vi "CRYChannel Table.vi"(1 "I_Device Info":T3(array[cluster]), 2 "I_Channel Info":T4[](array[typedef]) {"Coupling" items=["Default"=-1, "RSE"=10083, "NRSE"=10078, "Differential"=10106, "Pseudodifferential"=12529]; "term config" items=["Default"=-1, "RSE"=10083, "NRSE"=10078, "Differential"=10106, "Pseudodifferential"=12529]; "Anti-aliasing Factor (%fs)" format="%.2f"}, 7 "I_Name In":string[][](array[string]), 9 "O_Name In":string[][](array[string]), 12 "O_Device Info":T3(array[cluster]), 13 "O_Channel Info":T4[](array[typedef]) {"Coupling" items=["Default"=-1, "RSE"=10083, "NRSE"=10078, "Differential"=10106, "Pseudodifferential"=12529]; "term config" items=["Default"=-1, "RSE"=10083, "NRSE"=10078, "Differential"=10106, "Pseudodifferential"=12529]; "Anti-aliasing Factor (%fs)" format="%.2f"}) -> (4 "O_Channel Info Out":T4[](array[typedef]) {"Coupling" items=["Default"=-1, "RSE"=10083, "NRSE"=10078, "Differential"=10106, "Pseudodifferential"=12529]; "term config" items=["Default"=-1, "RSE"=10083, "NRSE"=10078, "Differential"=10106, "Pseudodifferential"=12529]; "Anti-aliasing Factor (%fs)" format="%.2f"}, 6 "I_Channel Info Out":T4[](array[typedef]) {"Coupling" items=["Default"=-1, "RSE"=10083, "NRSE"=10078, "Differential"=10106, "Pseudodifferential"=12529]; "term config" items=["Default"=-1, "RSE"=10083, "NRSE"=10078, "Differential"=10106, "Pseudodifferential"=12529]; "Anti-aliasing Factor (%fs)" format="%.2f"}, 8 "I_Name Out":string[][](array[string]), 10 "O_Name Out":string[][](array[string]), 15 "Return Flag":bool)   [LabVIEW 2013]
uses:
  Typedef Control/CRYHardware Channel Info.ctl
  <vilib>/Utility/miscctls.llb/LVBoundsTypeDef.ctl
  <vilib>/Utility/miscctls.llb/LVPositionTypeDef.ctl
  <vilib>/Utility/miscctls.llb/LVStringsAndValuesArrayTypeDef.ctl
panel:
  in  "Out_In Old":bool
  out "Row Old":i32
  out "Column Old":i32
  in  "Update":bool
  out "SelectValue":u32
  out "Device Name":string
  out "Cell Position":T1
  out "Cell Size":T2
  out "Column":i32
  out "Row":i32
  in  "Out_In":bool
  in  "SelectSate":bool
  in  "VmaxText":string
  in  "SelectRing":u32(ring) items=["8 bit"=8, "16 bit"=16, "24 bit"=24, "32 bit"=32]
  in  "I_MList":i32(listbox) caption="Input Channels"
  in  "I_Duplicate":bool
  in  "I_Delete":bool
  in  "I_Add":bool
  in  "O_Duplicate":bool
  in  "O_Delete":bool
  in  "O_Add":bool
  in  "Cancel":bool
  in  "OK":bool
  in  "O_MList":i32[](listbox) caption="Output Channels"
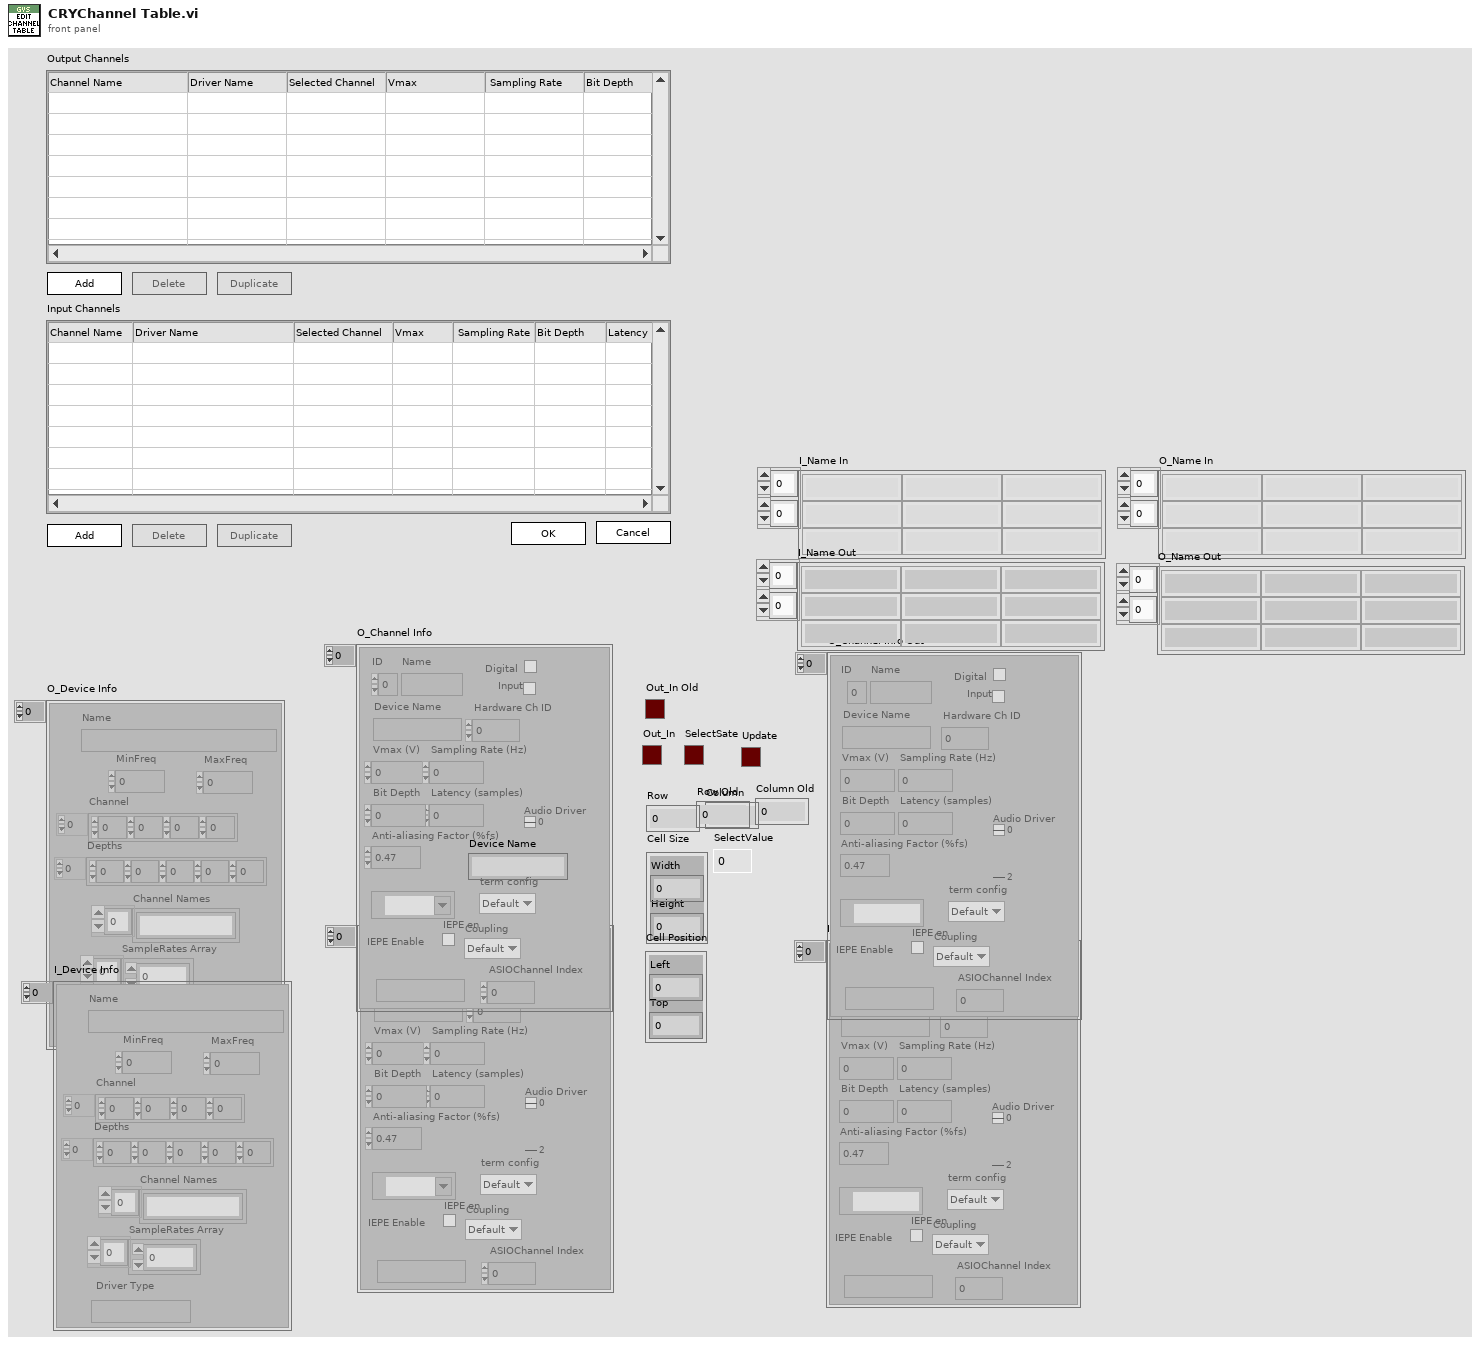
[diagram p1: front panel]
types:
  T1 = typedef "LVPositionTypeDef.ctl" = cluster{"Left":i32, "Top":i32}
  T2 = typedef "LVBoundsTypeDef.ctl" = cluster{"Width":u32, "Height":u32}
  T3 = cluster{"Name":string, "MinFreq":dbl, "MaxFreq":dbl, "Channel":i32[], "Depths":i32[], "Channel Names":string[], "SampleRates Array":dbl[], "Driver Type":string}[]
  T4 = typedef "CRYHardware Channel Info.ctl" = cluster{"ID":i32, "Name":string, "Digital":bool, "Input":bool, "Device Name":string, "Hardware Ch ID":u8, "Vmax (V)":dbl, "Latency (samples)":dbl, "Sampling Rate (Hz)":u32, "Bit Depth":u32, "Anti-aliasing Factor (%fs)":sgl, "DAQmx Channel":tag, "term config":i32, "Coupling":i32, "IEPE en":bool, "ASIOChannel Name":string, "Audio Driver":u16, "ASIOChannel Index":u8}
  T5 = typedef "LVStringsAndValuesArrayTypeDef.ctl" = cluster{"String":string, "Value":ext}[]
  T6 = typedef "LVPoint32TypeDef.ctl" = cluster{"Horizontal":i32, "Vertical":i32}
  T7 = typedef "LVRowAndColumnTypeDef.ctl" = cluster{"Row":i32, "Column":i32}
  T8 = cluster{"Name":string, "MinFreq":dbl, "MaxFreq":dbl, "Channel":i32[], "Depths":i32[], "Channel Names":string[], "SampleRates Array":dbl[], "Driver Type":string}
  T9 = cluster{"O_Add":bool, "O_Delete":bool, "O_Duplicate":bool, "I_Add":bool, "I_Delete":bool, "I_Duplicate":bool, "Update":bool}
  T10 = cluster{"Name":string, "Device Name":string, "Device Name":string, string, string, string}
  T11 = cluster{"Name":string, "Device Name":string, "Device Name":string, string, string, string, string}
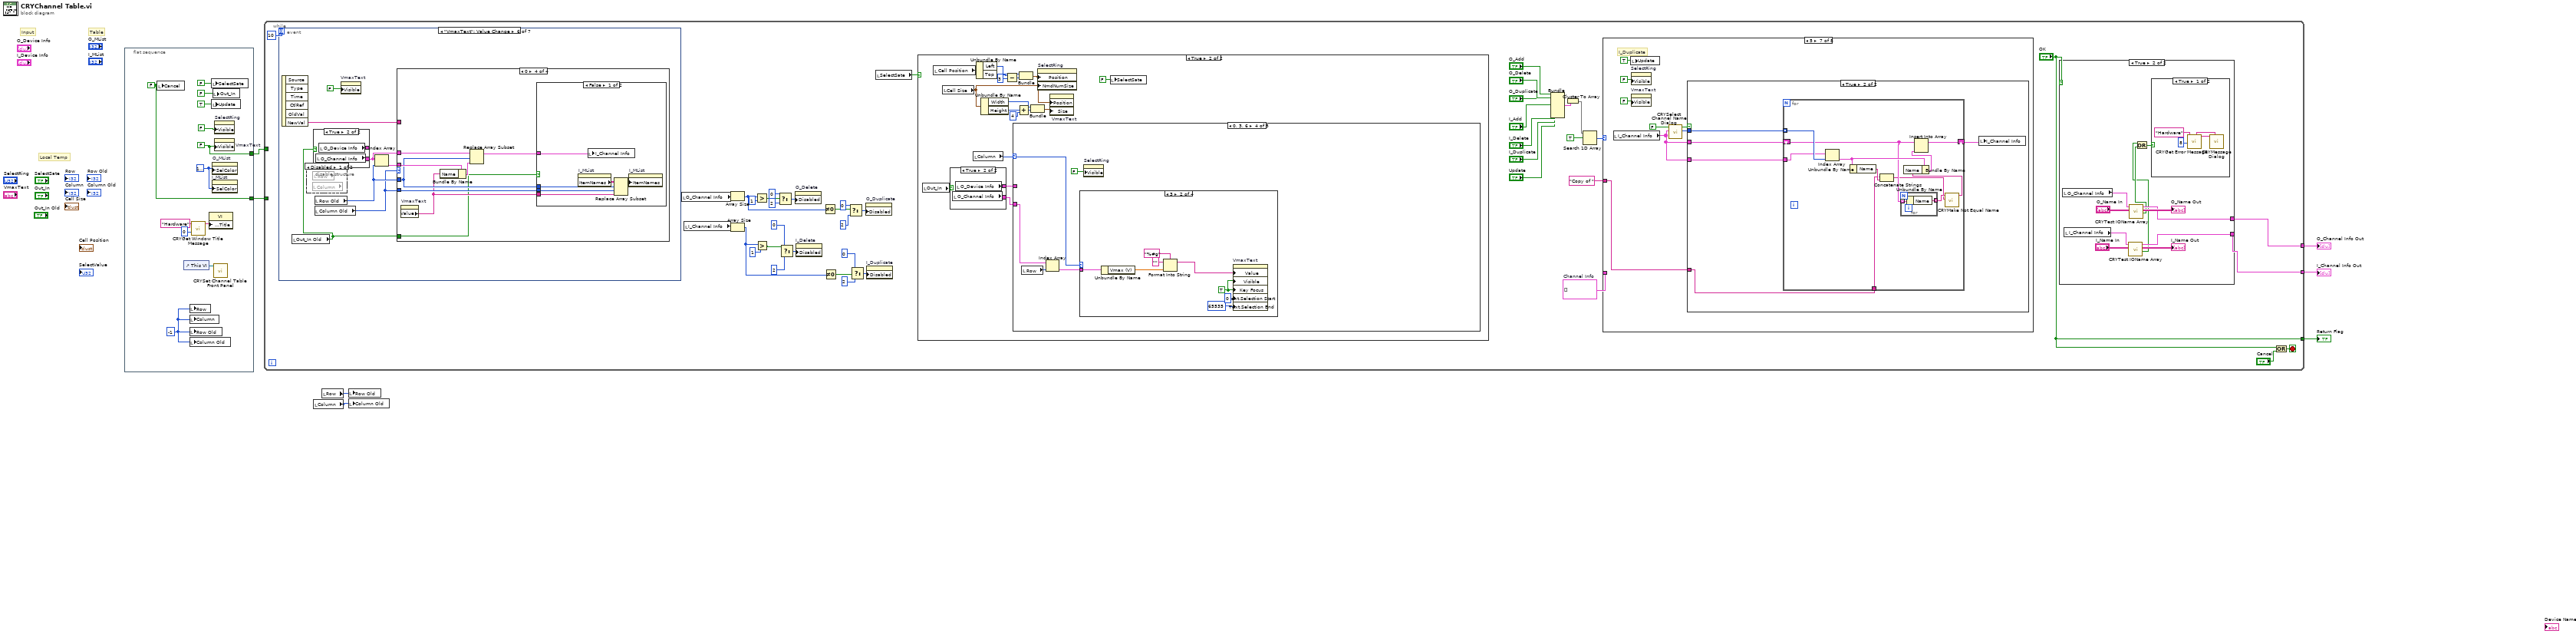
[diagram p0: block diagram]
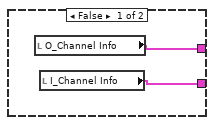
[diagram p2: hidden frame]
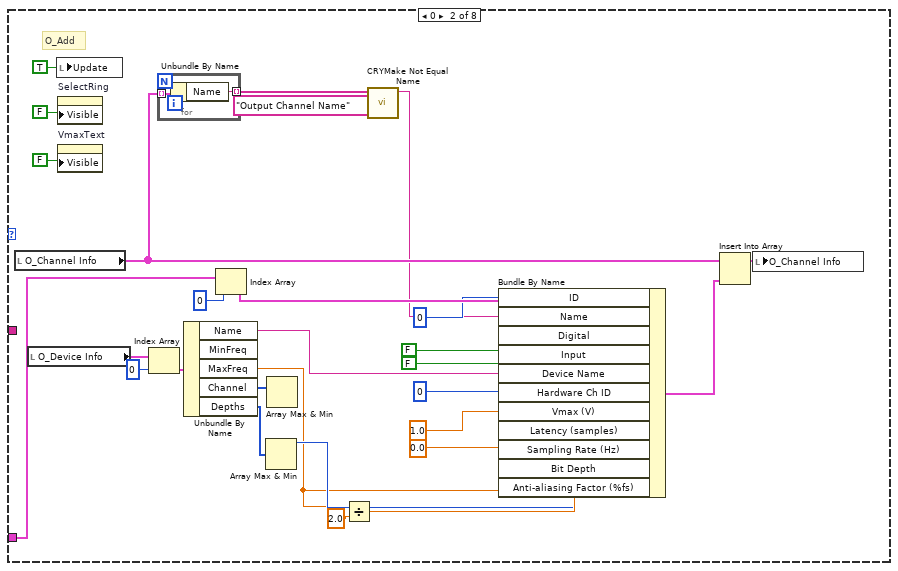
[diagram p5: hidden frame]
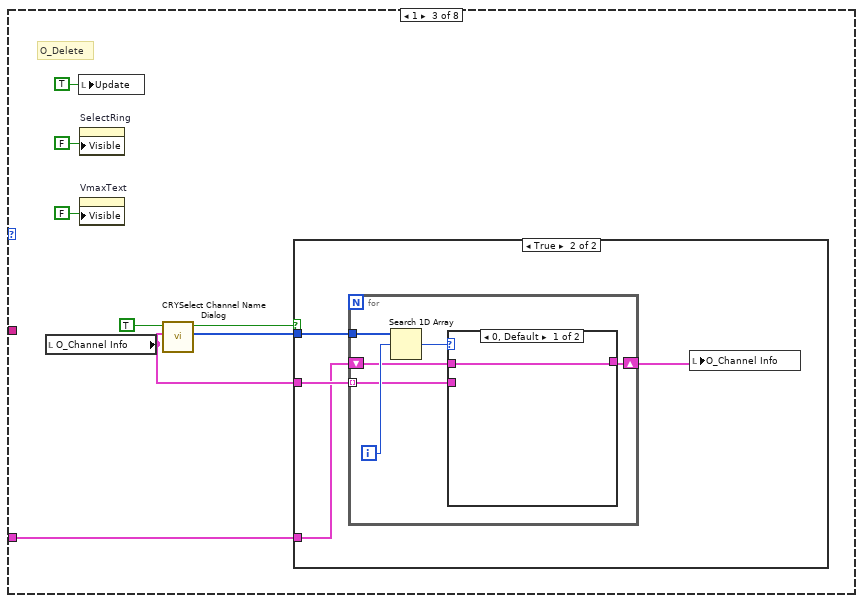
[diagram p6: hidden frame]
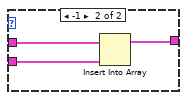
[diagram p8: hidden frame]
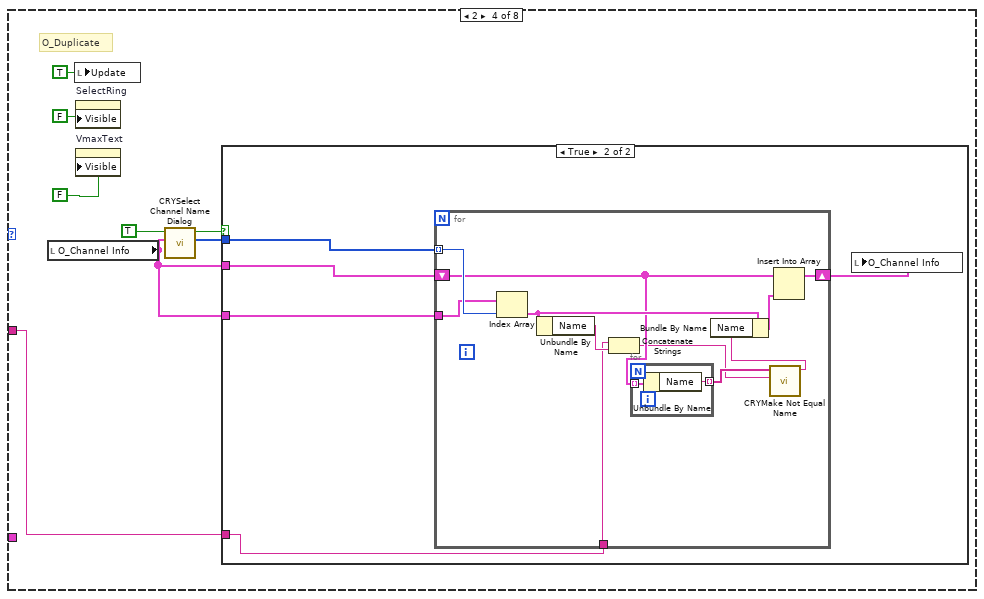
[diagram p9: hidden frame]
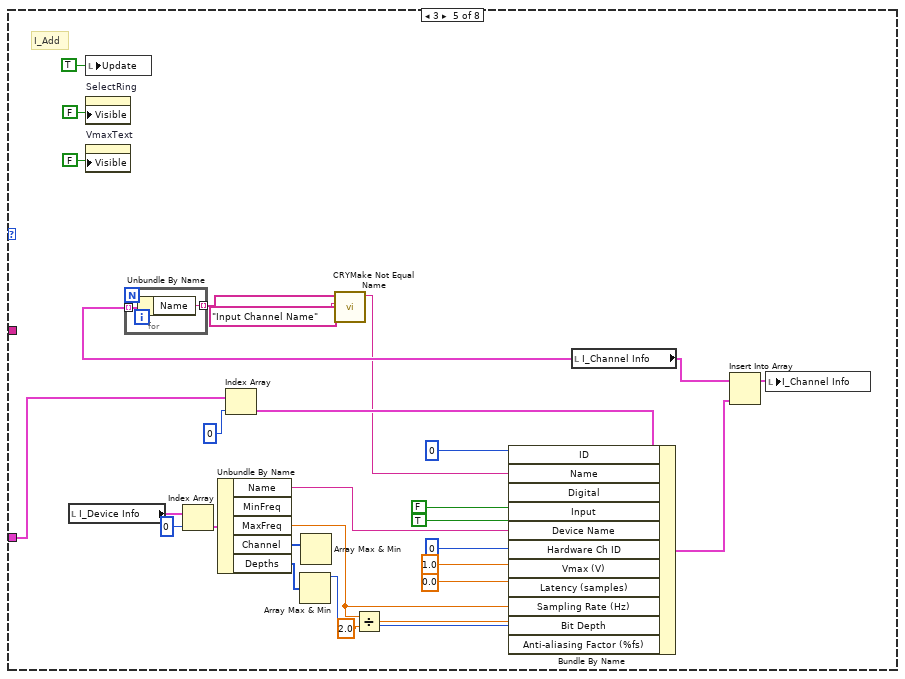
[diagram p11: hidden frame]
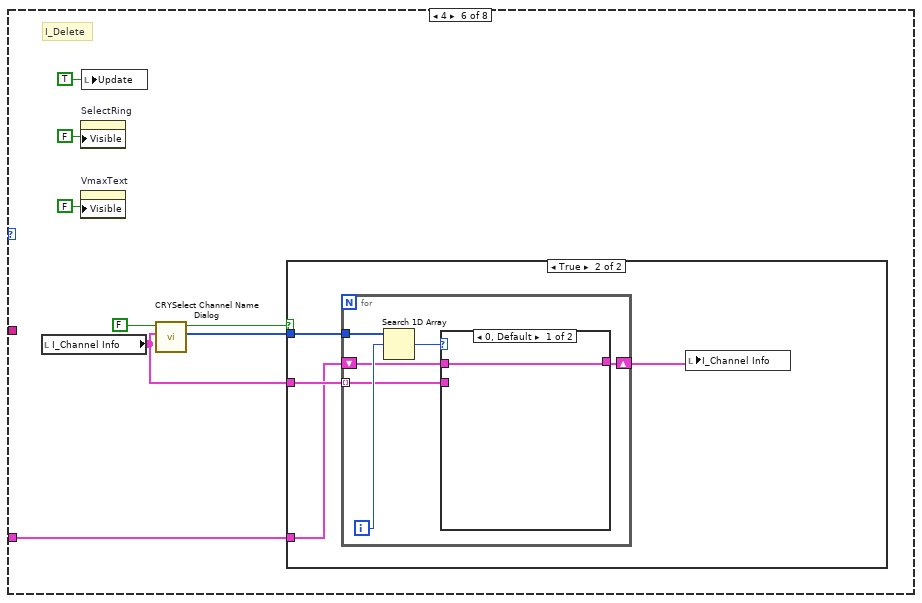
[diagram p12: hidden frame]
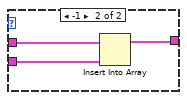
[diagram p14: hidden frame]
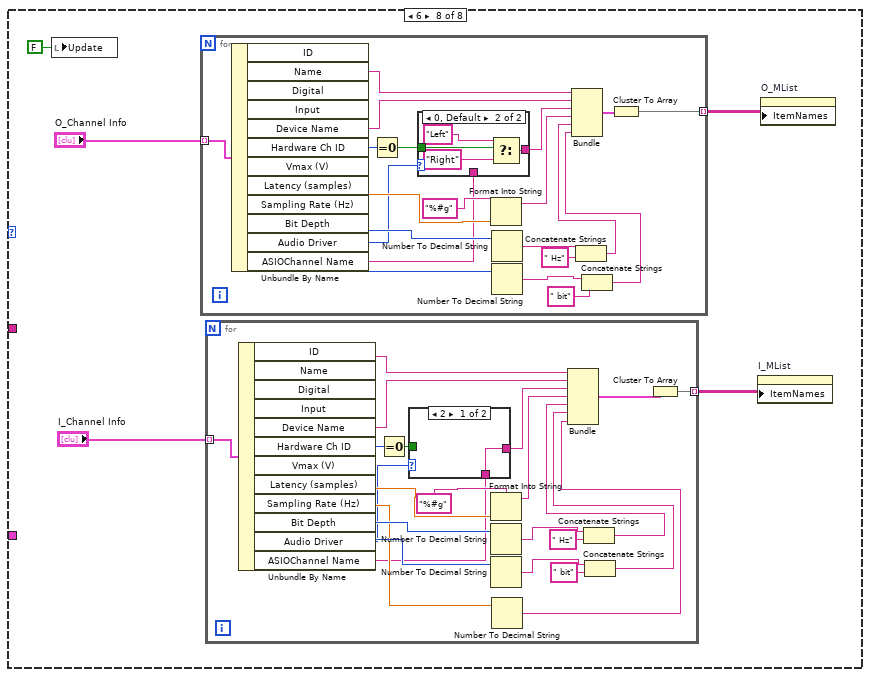
[diagram p16: hidden frame]
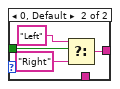
[diagram p17: hidden frame]
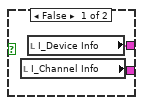
[diagram p20: hidden frame]
diagram:
  # "Table"
  # "Input"
  # "Local Temp"
  n1 = flat-sequence {
    tunnel: [w14] -> w4
    tunnel: [w9] -> w3
    frame #0 {
      w8 = -1 ("Row Old")
      w9 = FALSE ("Cancel")
      w15 = u32 16777226
      w14 = FALSE ("Visible")
      n2 = local write "Cancel"(w9) -> ()
      n3 = control-ref of="This VI"() -> (w10:refnum<vi>)
      n4 = local write "Row"(w8) -> ()
      n5 = local write "Column"(w8) -> ()
      n6 = local write "Row Old"(w8) -> ()
      n7 = local write "Column Old"(w8) -> ()
      n8 = call "CRYGet Window Title Message.vi"("No"=0 ("Error No"), "Kind"="Hardware") -> ("Multibyte String"=w13:string)  [unwired: 4 in, 5 out]
      n9 = property class="VI"("Front Panel.Title"=w13) -> ()  [unwired: 2 in, 2 out]
      n10 = local write "SelectSate"(FALSE ("SelectSate")) -> ()
      n11 = local write "Update"(TRUE ("Update")) -> ()
      n12 = property on="O_MList" class="MCListbox (strict)"("SelColor"=w15) -> ()  [unwired: 2 in, 2 out]
      n13 = property on="I_MList" class="MCListbox (strict)"("SelColor"=w15) -> ()  [unwired: 2 in, 2 out]
      n14 = local write "Out_In"(FALSE ("Out/In")) -> ()
      n15 = call "CRYSet Channel Table Front Panel.vi"("Vi Ref"=w10) -> ()  [unwired: 11 in]
      n16 = property on="SelectRing" class="Ring (strict)"("Visible"=FALSE) -> ()  [unwired: 2 in, 2 out]
      n17 = property on="VmaxText" class="Str"("Visible"=w14) -> ()  [unwired: 2 in, 2 out]
    }
  }
  n18 = while {
    tunnel: ["OK"] -> w7
    tunnel: [w21] -> w6
    tunnel: [w20] -> w5
    tunnel: w4 -> [_]
    tunnel: w3 -> [_]
    stop <- w61 stop-if-true
    w47 = T4[] []  # Channel Info
    n19 = event shown="[5] \"VmaxText\": Value Change" {
      selector: _ -> [_ _ _ _ _ _ _]
      dyn-events: _ -> [_ _ _ _ _ _ _]
      timeout: 10 -> [_ _ _ _ _ _ _]
      event Timeout {
        n20 = event-data() -> ()  [unwired: 3 out]
      }
      event "O_MList": Mouse Down {
        n21 = event-data() -> ("Coords"=w484:T6)  [unwired: 8 out]
        n22 = flat-sequence {
          tunnel: w477 -> [w497]
          tunnel: [w497] -> w476
          frame #0 {
            n23 = local read "Column"() -> (w499:i32)
            n24 = local read "Row"() -> (w498:i32)
            n25 = local write "Row Old"(w498) -> ()
            n26 = local write "Column Old"(w499) -> ()
          }
        }
        n27 = invoke on="O_MList" class="MCListbox (strict)" method="Point To Row Column"("Point"=w484) -> ("CellPosition"=w477:T7)  [unwired: 6 in, 6 out]
        n28 = local read "Row"() -> (w475:i32)
        n29 = case shown="0, Default" w475 {
          frame 0, Default {
            n30 = flat-sequence {
              frame #0 {
                n31 = local read "Out_In"() -> (w494:bool)
                n32 = local write "Out_In Old"(w494) -> ()
              }
              frame #1 {
                n33 = local write "Out_In"(TRUE ("Out/In")) -> ()
              }
            }
          }
          frame -1 {
            w496 = TRUE ("Out/In")
            n34 = local write "Out_In"(w496) -> ()
            n35 = local write "Out_In Old"(w496) -> ()
          }
        }
        n36 = property on="O_MList" class="MCListbox (strict)"("ActiveCell"=w476) -> ("CellSize"=w481:T2, "ActiveCellPos"=w482:T1)  [unwired: 2 in, 2 out]
        n37 = Unbundle By Name(w476) -> ("Row"=w479:i32, "Column"=w480:i32)
        n38 = local read "O_Channel Info"() -> (w493:T4[])
        n39 = local write "Cell Size"(w481) -> ()
        n40 = local write "Cell Position"(w482) -> ()
        n41 = Equal To 0?(x=w479) -> (x = 0?=w486:bool)
        n42 = Equal To 0?(x=w480) -> (x = 0?=w485:bool)
        n43 = local write "Row"(w479) -> ()
        n44 = local write "Column"(w480) -> ()
        n45 = Compound Arithmetic op=AND(w486, w485) -> (w478:bool)
        n46 = Array Size(array=w493) -> (size(s)=w492:i32)
        n47 = case shown="True" w478 {
          tunnel: w482 -> [_ w514]
          tunnel: w484 -> [_ w515]
          tunnel: w481 -> [_ w513]
          tunnel: [TRUE w501] -> w483
          frame False {
          }
          frame True {
            n48 = Unbundle By Name(w515) -> ("Horizontal"=w506:i32, "Vertical"=w510:i32)
            n49 = Unbundle By Name(w513) -> ("Width"=w512:u32, "Height"=w511:u32)
            n50 = Unbundle By Name(w514) -> ("Left"=w504:i32, "Top"=w502:i32)
            n51 = Add(x=w504, y=w512) -> (x+y=w505:u32)
            n52 = Add(x=w502, y=w511) -> (x+y=w503:u32)
            n53 = In Range and Coerce(upper limit=w505, x=w506, lower limit=w504) -> (In Range?=w509:bool)  [unwired: 1 out]
            n54 = In Range and Coerce(upper limit=w503, x=w510, lower limit=w502) -> (In Range?=w508:bool)  [unwired: 1 out]
            n55 = Compound Arithmetic op=AND(w509, w508) -> (w507:bool)
            n56 = case shown="True" w507 {
              tunnel: [FALSE TRUE] -> w501
              frame False {
              }
              frame True {
              }
            }
          }
        }
        n57 = Less?(x=w479, y=w492) -> (x < y?=w491:bool)
        n58 = Greater Or Equal?(x=w479, y=0) -> (x >= y?=w490:bool)
        n59 = Build Array(w491, w490, w483) -> (w489:bool[])
        n60 = And Array Elements(Boolean array=w489) -> (logical AND=w488:bool)
        n61 = local write "SelectSate"(w488) -> ()
        n62 = case shown="False" w488 {
          frame False {
            n63 = property on="VmaxText" class="Str"("Visible"=FALSE) -> ()  [unwired: 2 in, 2 out]
            n64 = property on="SelectRing" class="Ring (strict)"("Visible"=FALSE) -> ()  [unwired: 2 in, 2 out]
          }
          frame True {
          }
        }
      }
      event "O_MList", "I_MList": Mouse Move {
        n65 = event-data() -> ("Coords"=w528:T6)  [unwired: 5 out]
        n66 = invoke on="O_MList" class="MCListbox (strict)" method="Point To Row Column"("Point"=w528) -> ("CellPosition"=w527:T7)  [unwired: 6 in, 6 out]
        n67 = Unbundle By Name(w527) -> ("Row"=w524:i32, "Column"=w526:i32)
        n68 = local read "Column"() -> (w525:i32)
        n69 = local read "Row"() -> (w523:i32)
        n70 = Not Equal?(x=w526, y=w525) -> (x != y?=w521:bool)
        n71 = Not Equal?(x=w524, y=w523) -> (x != y?=w522:bool)
        n72 = Or(x=w522, y=w521) -> (x .or. y?=w520:bool)
        n73 = case shown="True" w520 {
          frame True {
            n74 = property on="SelectRing" class="Ring (strict)"("Visible"=FALSE) -> ()  [unwired: 2 in, 2 out]
          }
          frame False {
          }
        }
      }
      event "I_MList": Mouse Down {
        n75 = event-data() -> ("Coords"=w533:T6)  [unwired: 8 out]
        n76 = flat-sequence {
          tunnel: w532 -> [w553]
          tunnel: [w553] -> w531
          frame #0 {
            n77 = local read "Column"() -> (w555:i32)
            n78 = local read "Row"() -> (w554:i32)
            n79 = local write "Row Old"(w554) -> ()
            n80 = local write "Column Old"(w555) -> ()
          }
        }
        n81 = invoke on="I_MList" class="MCListbox (strict)" method="Point To Row Column"("Point"=w533) -> ("CellPosition"=w532:T7)  [unwired: 6 in, 6 out]
        n82 = local read "Row"() -> (w530:i32)
        n83 = local read "I_Channel Info"() -> (w549:T4[])
        n84 = property on="I_MList" class="MCListbox (strict)"("ActiveCell"=w531) -> ("CellSize"=w538:T2, "ActiveCellPos"=w539:T1)  [unwired: 2 in, 2 out]
        n85 = Unbundle By Name(w531) -> ("Row"=w535:i32, "Column"=w536:i32)
        n86 = case shown="0, Default" w530 {
          frame 0, Default {
            n87 = flat-sequence {
              frame #0 {
                n88 = local read "Out_In"() -> (w550:bool)
                n89 = local write "Out_In Old"(w550) -> ()
              }
              frame #1 {
                n90 = local write "Out_In"(FALSE ("Out/In")) -> ()
              }
            }
          }
          frame -1 {
            w552 = FALSE ("Out/In")
            n91 = local write "Out_In"(w552) -> ()
            n92 = local write "Out_In Old"(w552) -> ()
          }
        }
        n93 = Equal To 0?(x=w535) -> (x = 0?=w541:bool)
        n94 = Equal To 0?(x=w536) -> (x = 0?=w540:bool)
        n95 = local write "Column"(w536) -> ()
        n96 = local write "Cell Position"(w539) -> ()
        n97 = local write "Row"(w535) -> ()
        n98 = local write "Cell Size"(w538) -> ()
        n99 = Compound Arithmetic op=AND(w541, w540) -> (w534:bool)
        n100 = Array Size(array=w549) -> (size(s)=w548:i32)
        n101 = Less?(x=w535, y=w548) -> (x < y?=w545:bool)
        n102 = Greater Or Equal?(x=w535, y=0) -> (x >= y?=w544:bool)
        n103 = Greater Or Equal?(x=w536, y=1) -> ()  [unwired: 1 out]
        n104 = case shown="True" w534 {
          tunnel: w539 -> [_ w570]
          tunnel: w533 -> [_ w571]
          tunnel: w538 -> [_ w569]
          tunnel: [TRUE w557] -> w537
          frame False {
          }
          frame True {
            n105 = Unbundle By Name(w571) -> ("Horizontal"=w562:i32, "Vertical"=w566:i32)
            n106 = Unbundle By Name(w569) -> ("Width"=w568:u32, "Height"=w567:u32)
            n107 = Unbundle By Name(w570) -> ("Left"=w560:i32, "Top"=w558:i32)
            n108 = Add(x=w560, y=w568) -> (x+y=w561:u32)
            n109 = Add(x=w558, y=w567) -> (x+y=w559:u32)
            n110 = In Range and Coerce(upper limit=w561, x=w562, lower limit=w560) -> (In Range?=w565:bool)  [unwired: 1 out]
            n111 = In Range and Coerce(upper limit=w559, x=w566, lower limit=w558) -> (In Range?=w564:bool)  [unwired: 1 out]
            n112 = Compound Arithmetic op=AND(w565, w564) -> (w563:bool)
            n113 = case shown="False" w563 {
              tunnel: [FALSE TRUE] -> w557
              frame False {
              }
              frame True {
              }
            }
          }
        }
        n114 = Build Array(w545, w544, w537) -> (w543:bool[])
        n115 = And Array Elements(Boolean array=w543) -> (logical AND=w542:bool)
        n116 = case shown="False" w542 {
          frame False {
            n117 = property on="VmaxText" class="Str"("Visible"=FALSE) -> ()  [unwired: 2 in, 2 out]
            n118 = property on="SelectRing" class="Ring (strict)"("Visible"=FALSE) -> ()  [unwired: 2 in, 2 out]
          }
          frame True {
          }
        }
        n119 = local write "SelectSate"(w542) -> ()
      }
      event "SelectRing": Value Change {
        n120 = event-data() -> ("NewVal"=w578:u32)  [unwired: 6 out]
        n121 = local read "Out_In"() -> (w583:bool)
        n122 = case shown="False" w583 {
          tunnel: [w699 w701] -> w579
          tunnel: [w698 w700] -> w580
          frame False {
            n123 = local read "I_Channel Info"() -> (w699:T4[])
            n124 = local read "I_Device Info"() -> (w698:T3)
          }
          frame True {
            n125 = local read "O_Channel Info"() -> (w701:T4[])
            n126 = local read "O_Device Info"() -> (w700:T3)
          }
        }
        n127 = local write "Update"(TRUE ("Update")) -> ()
        n128 = local read "Column"() -> (w582:i32)
        n129 = local read "Row"() -> (w577:i32)
        n130 = Index Array(array=w579, index=w577) -> (element=w581:T4)
        n131 = case shown="1" w582 {
          selector: w582 -> [_ w596 w637 w658 w678]
          tunnel: w581 -> [_ w588 w639 w663 w679]
          tunnel: w580 -> [_ w590 _ _ _]
          tunnel: w579 -> [_ w595 w640 w664 w680]
          tunnel: w578 -> [_ w593 w636 w662 w681]
          tunnel: w577 -> [_ w594 w638 w659 w677]
          frame 0, Default {
          }
          frame 1 {
            n132 = Unbundle By Name(w588) -> ("Audio Driver"=w587:u16)
            n133 = case shown="0, Default" w587 {
              tunnel: w590 -> [w603 w614]
              tunnel: [w602 w613] -> w589
              frame 2 {
                n134 = for {
                  tunnel: w603 -> [w604] mode=indexing
                  shift-right: [w606] -> w602
                  shift-left: T3 [] -> [w605]
                  n135 = Unbundle By Name(w604) -> ("Driver Type"=w607:string)
                  n136 = case shown="\"ASIO\"" w607 {
                    tunnel: [w608 w611] -> w606
                    tunnel: w605 -> [w608 w610]
                    tunnel: w604 -> [_ w609]
                    frame "False", Default {
                    }
                    frame "ASIO" {
                      n137 = Build Array (concatenate)(w610, w609) -> (w611:T3)
                    }
                  }
                }
              }
              frame 0, Default {
                n138 = for {
                  tunnel: w614 -> [w615] mode=indexing
                  shift-right: [w617] -> w613
                  shift-left: T3 [] -> [w616]
                  n139 = Unbundle By Name(w615) -> ("Driver Type"=w618:string)
                  n140 = case shown="\"MME\"" w618 {
                    tunnel: [w619 w622] -> w617
                    tunnel: w616 -> [w619 w621]
                    tunnel: w615 -> [_ w620]
                    frame "False", Default {
                    }
                    frame "MME" {
                      n141 = Build Array (concatenate)(w621, w620) -> (w622:T3)
                    }
                  }
                }
              }
            }
            n142 = Index Array(array=w589, index=w593) -> (element=w592:T8)
            n143 = Unbundle By Name(w592) -> ("Channel Names"=w585:string[], "Name"=w591:string)
            n144 = property on="SelectRing" class="Ring (strict)"() -> ("RingText.Text"=w598:string)  [unwired: 2 in, 2 out]
            n145 = local read "Out_In"() -> (w597:bool)
            n146 = Index Array(array=w585) -> (element=w584:string)  [unwired: 1 in]
            n147 = Bundle By Name(cluster=w588, "Device Name"=w591, "Hardware Ch ID"=u8 0, "ASIOChannel Name"=w584) -> (w600:T4)
            n148 = Replace Array Subset(array=w595, new element=w600, index=w594) -> (w599:T4[])
            n149 = case shown="False" w597 {
              tunnel: w599 -> [w628 w634]
              tunnel: w594 -> [w627 w632]
              tunnel: w596 -> [w626 w631]
              tunnel: w598 -> [w625 w630]
              frame False {
                n150 = property on="I_MList" class="MCListbox (strict)"() -> ("ItemNames"=w624:string[][])  [unwired: 2 in, 2 out]
                n151 = local write "I_Channel Info"(w628) -> ()
                n152 = Replace Array Subset(array=w624, new element=w625, index (row)=w627, index (col)=w626) -> (w623:string[][])
                n153 = property on="I_MList" class="MCListbox (strict)"("ItemNames"=w623) -> ()  [unwired: 2 in, 2 out]
              }
              frame True {
                n154 = local write "O_Channel Info"(w634) -> ()
                n155 = property on="O_MList" class="MCListbox (strict)"() -> ("ItemNames"=w633:string[][])  [unwired: 2 in, 2 out]
                n156 = Replace Array Subset(array=w633, new element=w630, index (row)=w632, index (col)=w631) -> (w629:string[][])
                n157 = property on="O_MList" class="MCListbox (strict)"("ItemNames"=w629) -> ()  [unwired: 2 in, 2 out]
              }
            }
          }
          frame 2 {
            n158 = property on="SelectRing" class="Ring (strict)"() -> ("RingText.Text"=w635:string)  [unwired: 2 in, 2 out]
            n159 = Bundle By Name(cluster=w639, "Hardware Ch ID"=w636, "ASIOChannel Name"=w635) -> (w643:T4)
            n160 = local read "Out_In"() -> (w641:bool)
            n161 = Replace Array Subset(array=w640, new element=w643, index=w638) -> (w642:T4[])
            n162 = case shown="False" w641 {
              tunnel: w642 -> [w649 w655]
              tunnel: w638 -> [w648 w653]
              tunnel: w637 -> [w647 w652]
              tunnel: w635 -> [w646 w651]
              frame False {
                n163 = property on="I_MList" class="MCListbox (strict)"() -> ("ItemNames"=w645:string[][])  [unwired: 2 in, 2 out]
                n164 = local write "I_Channel Info"(w649) -> ()
                n165 = Replace Array Subset(array=w645, new element=w646, index (row)=w648, index (col)=w647) -> (w644:string[][])
                n166 = property on="I_MList" class="MCListbox (strict)"("ItemNames"=w644) -> ()  [unwired: 2 in, 2 out]
              }
              frame True {
                n167 = local write "O_Channel Info"(w655) -> ()
                n168 = property on="O_MList" class="MCListbox (strict)"() -> ("ItemNames"=w654:string[][])  [unwired: 2 in, 2 out]
                n169 = Replace Array Subset(array=w654, new element=w651, index (row)=w653, index (col)=w652) -> (w650:string[][])
                n170 = property on="O_MList" class="MCListbox (strict)"("ItemNames"=w650) -> ()  [unwired: 2 in, 2 out]
              }
            }
          }
          frame 4 {
            n171 = Bundle By Name(cluster=w663, "Sampling Rate (Hz)"=w662) -> (w661:T4)
            n172 = property on="SelectRing" class="Ring (strict)"() -> ("RingText.Text"=w657:string)  [unwired: 2 in, 2 out]
            n173 = local read "Out_In"() -> (w656:bool)
            n174 = Replace Array Subset(array=w664, new element=w661, index=w659) -> (w660:T4[])
            n175 = case shown="False" w656 {
              tunnel: w660 -> [w670 w676]
              tunnel: w659 -> [w669 w674]
              tunnel: w658 -> [w668 w673]
              tunnel: w657 -> [w667 w672]
              frame False {
                n176 = property on="I_MList" class="MCListbox (strict)"() -> ("ItemNames"=w666:string[][])  [unwired: 2 in, 2 out]
                n177 = local write "I_Channel Info"(w670) -> ()
                n178 = Replace Array Subset(array=w666, new element=w667, index (row)=w669, index (col)=w668) -> (w665:string[][])
                n179 = property on="I_MList" class="MCListbox (strict)"("ItemNames"=w665) -> ()  [unwired: 2 in, 2 out]
              }
              frame True {
                n180 = local write "O_Channel Info"(w676) -> ()
                n181 = property on="O_MList" class="MCListbox (strict)"() -> ("ItemNames"=w675:string[][])  [unwired: 2 in, 2 out]
                n182 = Replace Array Subset(array=w675, new element=w672, index (row)=w674, index (col)=w673) -> (w671:string[][])
                n183 = property on="O_MList" class="MCListbox (strict)"("ItemNames"=w671) -> ()  [unwired: 2 in, 2 out]
              }
            }
          }
          frame 5 {
            n184 = Bundle By Name(cluster=w679, "Bit Depth"=w681) -> (w685:T4)
            n185 = property on="SelectRing" class="Ring (strict)"() -> ("RingText.Text"=w683:string)  [unwired: 2 in, 2 out]
            n186 = local read "Out_In"() -> (w682:bool)
            n187 = Replace Array Subset(array=w680, new element=w685, index=w677) -> (w684:T4[])
            n188 = case shown="False" w682 {
              tunnel: w684 -> [w691 w697]
              tunnel: w677 -> [w690 w695]
              tunnel: w678 -> [w689 w694]
              tunnel: w683 -> [w688 w693]
              frame False {
                n189 = property on="I_MList" class="MCListbox (strict)"() -> ("ItemNames"=w687:string[][])  [unwired: 2 in, 2 out]
                n190 = local write "I_Channel Info"(w691) -> ()
                n191 = Replace Array Subset(array=w687, new element=w688, index (row)=w690, index (col)=w689) -> (w686:string[][])
                n192 = property on="I_MList" class="MCListbox (strict)"("ItemNames"=w686) -> ()  [unwired: 2 in, 2 out]
              }
              frame True {
                n193 = local write "O_Channel Info"(w697) -> ()
                n194 = property on="O_MList" class="MCListbox (strict)"() -> ("ItemNames"=w696:string[][])  [unwired: 2 in, 2 out]
                n195 = Replace Array Subset(array=w696, new element=w693, index (row)=w695, index (col)=w694) -> (w692:string[][])
                n196 = property on="O_MList" class="MCListbox (strict)"("ItemNames"=w692) -> ()  [unwired: 2 in, 2 out]
              }
            }
          }
        }
      }
      event "VmaxText": Value Change {
        n197 = event-data() -> ("NewVal"=w706:string)  [unwired: 6 out]
        n198 = local read "Out_In Old"() -> (w702:bool)
        n199 = disable-structure shown="Disabled" {
          frame Disabled {
            n200 = local read "Column"() -> ()  [unwired: 1 out]
            n201 = local read "Row"() -> ()  [unwired: 1 out]
          }
          frame Enabled {
          }
        }
        n202 = case shown="True" w702 {
          tunnel: [w772 w774] -> w707
          tunnel: [w771 w773] -> _
          frame False {
            n203 = local read "I_Channel Info"() -> (w772:T4[])
            n204 = local read "I_Device Info"() -> (w771:T3)
          }
          frame True {
            n205 = local read "O_Channel Info"() -> (w774:T4[])
            n206 = local read "O_Device Info"() -> (w773:T3)
          }
        }
        n207 = local read "Row Old"() -> (w704:i32)
        n208 = local read "Column Old"() -> (w703:i32)
        n209 = property on="VmaxText" class="Str"("Visible"=FALSE) -> ()  [unwired: 2 in, 2 out]
        n210 = Index Array(array=w707, index=w704) -> (element=w708:T4)
        n211 = case shown="0" w703 {
          tunnel: w703 -> [_ w721 w739 w758]
          tunnel: w708 -> [_ w720 w738 w757]
          tunnel: w707 -> [_ w719 w737 w756]
          tunnel: w704 -> [_ w718 w736 w755]
          tunnel: w706 -> [_ w715 w735 _]
          tunnel: w702 -> [_ w709 w734 w751]
          frame 1, Default {
          }
          frame 3 {
            n212 = Scan Value(string=w715, format string="%f") -> (value=w711:dbl)  [unwired: 1 in, 1 out]
            n213 = Bundle By Name(cluster=w720, "Vmax (V)"=w711) -> (w717:T4)
            n214 = Format Into String(format string="%#g", initial string="", w711) -> (resulting string=w710:string)  [unwired: 1 in, 1 out]
            n215 = Replace Array Subset(array=w719, new element=w717, index=w718) -> (w716:T4[])
            n216 = case shown="False" w709 {
              tunnel: w716 -> [w727 w733]
              tunnel: w718 -> [w726 w731]
              tunnel: w721 -> [w725 w730]
              tunnel: w710 -> [w724 w729]
              frame False {
                n217 = property on="I_MList" class="MCListbox (strict)"() -> ("ItemNames"=w723:string[][])  [unwired: 2 in, 2 out]
                n218 = local write "I_Channel Info"(w727) -> ()
                n219 = Replace Array Subset(array=w723, new element=w724, index (row)=w726, index (col)=w725) -> (w722:string[][])
                n220 = property on="I_MList" class="MCListbox (strict)"("ItemNames"=w722) -> ()  [unwired: 2 in, 2 out]
              }
              frame True {
                n221 = local write "O_Channel Info"(w733) -> ()
                n222 = property on="O_MList" class="MCListbox (strict)"() -> ("ItemNames"=w732:string[][])  [unwired: 2 in, 2 out]
                n223 = Replace Array Subset(array=w732, new element=w729, index (row)=w731, index (col)=w730) -> (w728:string[][])
                n224 = property on="O_MList" class="MCListbox (strict)"("ItemNames"=w728) -> ()  [unwired: 2 in, 2 out]
              }
            }
          }
          frame 6 {
            n225 = case shown="False" w734 {
              tunnel: w739 -> [_ w750]
              tunnel: w738 -> [_ w749]
              tunnel: w737 -> [_ w748]
              tunnel: w736 -> [_ w747]
              tunnel: w735 -> [_ w746]
              frame True {
              }
              frame False {
                n226 = Decimal String To Number(string=w746) -> (number=w743:i32)  [unwired: 3 out]
                n227 = Bundle By Name(cluster=w749, "Latency (samples)"=w743) -> (w745:T4)
                n228 = Number To Decimal String(number=w743) -> (decimal integer string=w742:string)  [unwired: 1 out]
                n229 = Replace Array Subset(array=w748, new element=w745, index=w747) -> (w744:T4[])
                n230 = property on="I_MList" class="MCListbox (strict)"() -> ("ItemNames"=w741:string[][])  [unwired: 2 in, 2 out]
                n231 = local write "I_Channel Info"(w744) -> ()
                n232 = Replace Array Subset(array=w741, new element=w742, index (row)=w747, index (col)=w750) -> (w740:string[][])
                n233 = property on="I_MList" class="MCListbox (strict)"("ItemNames"=w740) -> ()  [unwired: 2 in, 2 out]
              }
            }
          }
          frame 0 {
            n234 = property on="VmaxText" class="Str"() -> ("Value"=w752:string)  [unwired: 2 in, 2 out]
            n235 = Bundle By Name(cluster=w757, "Name"=w752) -> (w754:T4)
            n236 = Replace Array Subset(array=w756, new element=w754, index=w755) -> (w753:T4[])
            n237 = case shown="False" w751 {
              tunnel: w753 -> [w764 w770]
              tunnel: w755 -> [w759 w765]
              tunnel: w758 -> [w763 w768]
              tunnel: w752 -> [w760 w766]
              frame False {
                n238 = property on="I_MList" class="MCListbox (strict)"() -> ("ItemNames"=w762:string[][])  [unwired: 2 in, 2 out]
                n239 = local write "I_Channel Info"(w764) -> ()
                n240 = Replace Array Subset(array=w762, new element=w760, index (row)=w759, index (col)=w763) -> (w761:string[][])
                n241 = property on="I_MList" class="MCListbox (strict)"("ItemNames"=w761) -> ()  [unwired: 2 in, 2 out]
              }
              frame True {
                n242 = local write "O_Channel Info"(w770) -> ()
                n243 = property on="O_MList" class="MCListbox (strict)"() -> ("ItemNames"=w769:string[][])  [unwired: 2 in, 2 out]
                n244 = Replace Array Subset(array=w769, new element=w766, index (row)=w765, index (col)=w768) -> (w767:string[][])
                n245 = property on="O_MList" class="MCListbox (strict)"("ItemNames"=w767) -> ()  [unwired: 2 in, 2 out]
              }
            }
          }
        }
      }
      event Panel Close {
        n246 = event-data() -> ()  [unwired: 5 out]
        n247 = property on="Cancel" class="Bool (strict)"("Val(Sgnl)"=TRUE ("Update")) -> ()  [unwired: 2 in, 2 out]
      }
    }
    n248 = local read "O_Channel Info"() -> (w36:T4[])
    n249 = local read "I_Channel Info"() -> (w35:T4[])
    n250 = Array Size(array=w36) -> (size(s)=w33:i32)
    n251 = Array Size(array=w35) -> (size(s)=w32:i32)
    n252 = Greater?(x=w33, y=1) -> (0:w39:bool)
    n253 = Greater?(x=w32, y=1) -> (0:w46:bool)
    n254 = Select(t=u8 0, s=w39, f=u8 2) -> (s? t:f=w42:u8)
    n255 = Select(t=u8 0, s=w46, f=u8 2) -> (s? t:f=w45:u8)
    n256 = property on="O_Delete" class="Bool"("Disabled"=w42) -> ()  [unwired: 2 in, 2 out]
    n257 = property on="I_Delete" class="Bool"("Disabled"=w45) -> ()  [unwired: 2 in, 2 out]
    n258 = Not Equal To 0?(x=w33) -> (x != 0?=w24:bool)
    n259 = Not Equal To 0?(x=w32) -> (x != 0?=w25:bool)
    n260 = Select(t=u8 0, s=w24, f=u8 2) -> (s? t:f=w29:u8)
    n261 = Select(t=u8 0, s=w25, f=u8 2) -> (s? t:f=w26:u8)
    n262 = property on="O_Duplicate" class="Bool"("Disabled"=w29) -> ()  [unwired: 2 in, 2 out]
    n263 = property on="I_Duplicate" class="Bool"("Disabled"=w26) -> ()  [unwired: 2 in, 2 out]
    n264 = local read "SelectSate"() -> (w60:bool)
    n265 = case shown="True" w60 {
      frame False {
      }
      frame True {
        n266 = local read "Out_In"() -> (w304:bool)
        n267 = local read "Cell Position"() -> (w309:T1)
        n268 = local read "Cell Size"() -> (w299:T2)
        n269 = case shown="True" w304 {
          tunnel: [w312 w314] -> w303
          tunnel: [w311 w313] -> w302
          frame False {
            n270 = local read "I_Channel Info"() -> (w312:T4[])
            n271 = local read "I_Device Info"() -> (w311:T3)
          }
          frame True {
            n272 = local read "O_Channel Info"() -> (w314:T4[])
            n273 = local read "O_Device Info"() -> (w313:T3)
          }
        }
        n274 = local read "Column"() -> (w300:i32)
        n275 = Unbundle By Name(w309) -> ("Left"=w306:i32, "Top"=w307:i32)
        n276 = Unbundle By Name(w299) -> ("Width"=w297:u32, "Height"=w298:u32)
        n277 = Subtract(x=w307, y=3) -> (x-y=w305:i32)
        n278 = case shown="0, 3, 6" w300 {
          selector: w300 -> [_ _ _ w389 w420]
          tunnel: w303 -> [_ w320 w362 w391 w423]
          tunnel: w302 -> [_ w316 w358 _ w421]
          frame Default {
          }
          frame 1 {
            n279 = local read "Row"() -> (w321:i32)
            n280 = Index Array(array=w320, index=w321) -> (element=w322:T4)
            n281 = Unbundle By Name(w322) -> ("Device Name"=w319:string, "Audio Driver"=w317:u16)
            n282 = case shown="2" w317 {
              tunnel: w316 -> [w328 w339]
              tunnel: [w327 w338] -> w315
              frame 2 {
                n283 = for {
                  tunnel: w328 -> [w329] mode=indexing
                  shift-right: [w331] -> w327
                  shift-left: T3 [] -> [w330]
                  n284 = Unbundle By Name(w329) -> ("Driver Type"=w332:string)
                  n285 = case shown="\"ASIO\"" w332 {
                    tunnel: [w333 w336] -> w331
                    tunnel: w330 -> [w333 w335]
                    tunnel: w329 -> [_ w334]
                    frame "False", Default {
                    }
                    frame "ASIO" {
                      n286 = Build Array (concatenate)(w335, w334) -> (w336:T3)
                    }
                  }
                }
              }
              frame 0, Default {
                n287 = for {
                  tunnel: w339 -> [w340] mode=indexing
                  shift-right: [w342] -> w338
                  shift-left: T3 [] -> [w341]
                  n288 = Unbundle By Name(w340) -> ("Driver Type"=w343:string)
                  n289 = case shown="\"MME\"" w343 {
                    tunnel: [w344 w347] -> w342
                    tunnel: w341 -> [w344 w346]
                    tunnel: w340 -> [_ w345]
                    frame "False", Default {
                    }
                    frame "MME" {
                      n290 = Build Array (concatenate)(w346, w345) -> (w347:T3)
                    }
                  }
                }
              }
            }
            n291 = property on="VmaxText" class="Str"("Visible"=FALSE) -> ()  [unwired: 2 in, 2 out]
            n292 = for {
              tunnel: w315 -> [w355] mode=indexing
              shift-right: [w353] -> w323
              shift-left: cluster{"Name":string, i32}[] [] -> [w352]
              tunnel: w319 -> [w351]
              i -> [w349]
              n293 = Unbundle By Name(w355) -> ("Name"=w350:string)
              n294 = Bundle("Name"=w350, w349) -> (w354:cluster{"Name":string, i32})  [unwired: 1 out]
              n295 = Insert Into Array(array=w352, new element=w354) -> (w353:cluster{"Name":string, i32}[])  [unwired: 1 in]
              n296 = Equal?(x=w350, y=w351) -> (x = y?=w348:bool)
              n297 = case shown="True" w348 {
                tunnel: w349 -> [_ w356]
                frame False {
                }
                frame True {
                  n298 = property on="SelectRing" class="Ring (strict)"("Value"=w356) -> ()  [unwired: 2 in, 2 out]
                }
              }
            }
            n299 = property on="SelectRing" class="Ring (strict)"("StringsAndValues[]"=w323, "Visible"=TRUE) -> ()  [unwired: 2 in, 2 out]
          }
          frame 2 {
            n300 = local read "Row"() -> (w363:i32)
            n301 = Index Array(array=w362, index=w363) -> (element=w364:T4)
            n302 = Unbundle By Name(w364) -> ("Device Name"=w357:string, "Hardware Ch ID"=w361:u8, "Audio Driver"=w359:u16)
            n303 = property on="VmaxText" class="Str"("Visible"=FALSE) -> ()  [unwired: 2 in, 2 out]
            n304 = case shown="2" w359 {
              tunnel: w361 -> [w365 w386]
              tunnel: w358 -> [w372 _]
              tunnel: w357 -> [w373 _]
              frame 2 {
                n305 = call "CRYGet Device Index to Channel.vi"("Device Name In"=w373, "Device Info In"=w372) -> ("Device Index Out"=w369:i32)  [unwired: 9 out]
                n306 = for {
                  tunnel: w372 -> [w380] mode=indexing
                  shift-right: [w379] -> w370
                  shift-left: T3 [] -> [w378]
                  n307 = Unbundle By Name(w380) -> ("Driver Type"=w381:string)
                  n308 = case shown="\"ASIO\"" w381 {
                    tunnel: w380 -> [w384 _]
                    tunnel: [w383 w385] -> w379
                    tunnel: w378 -> [w382 w385]
                    frame "ASIO" {
                      n309 = Build Array (concatenate)(w382, w384) -> (w383:T3)
                    }
                    frame Default {
                    }
                  }
                }
                n310 = Index Array(array=w370, index=w369) -> (element=w368:T8)
                n311 = Unbundle By Name(w368) -> ("Channel Names"=w367:string[])
                n312 = for {
                  tunnel: w367 -> [w377] mode=indexing
                  tunnel: [w375] -> w366 mode=indexing
                  i -> [w376]
                  n313 = Bundle("return type"=w377, w376) -> (w375:cluster{"return type":string, i32})  [unwired: 1 in]
                }
                n314 = property on="SelectRing" class="Ring (strict)"("StringsAndValues[]"=w366, "Visible"=TRUE, "Value"=w365) -> ()  [unwired: 2 in, 2 out]
              }
              frame 0, Default {
                n315 = property on="SelectRing" class="Ring (strict)"("StringsAndValues[]"=T5 [{"String"="Left", "Value"=0.0}, {"String"="Right", "Value"=1.0}] ("Strings And Values []"), "Visible"=TRUE, "Value"=w386) -> ()  [unwired: 2 in, 2 out]
              }
            }
          }
          frame 0, 3, 6 {
            n316 = local read "Row"() -> (w392:i32)
            n317 = Index Array(array=w391, index=w392) -> (element=w393:T4)
            n318 = case shown="3" w389 {
              tunnel: w393 -> [_ w401 w403 w414]
              frame 1, Default {
              }
              frame 3 {
                w400 = TRUE ("Visible")
                n319 = Unbundle By Name(w401) -> ("Vmax (V)"=w395:dbl)
                n320 = Format Into String(format string="%#g", initial string="", w395) -> (resulting string=w394:string)  [unwired: 1 in, 1 out]
                n321 = property on="VmaxText" class="Str"("Value"=w394, "Visible"=w400, "Key Focus"=w400, "Text.Selection Start"=u32 0 ("Text.Selection:Start"), "Text.Selection End"=u32 65535 ("Text.Selection:End")) -> ()  [unwired: 2 in, 2 out]
              }
              frame 6 {
                n322 = local read "Out_In"() -> (w402:bool)
                n323 = case shown="False" w402 {
                  tunnel: w403 -> [_ w409]
                  frame True {
                  }
                  frame False {
                    w407 = TRUE ("Visible")
                    n324 = Unbundle By Name(w409) -> ("Latency (samples)"=w408:dbl)
                    n325 = Number To Decimal String(number=w408) -> (decimal integer string=w404:string)  [unwired: 1 out]
                    n326 = property on="VmaxText" class="Str"("Value"=w404, "Visible"=w407, "Key Focus"=w407, "Text.Selection Start"=u32 0 ("Text.Selection:Start"), "Text.Selection End"=u32 65535 ("Text.Selection:End")) -> ()  [unwired: 2 in, 2 out]
                  }
                }
              }
              frame 0 {
                w413 = TRUE ("Visible")
                n327 = Unbundle By Name(w414) -> ("Name"=w412:string)
                n328 = property on="VmaxText" class="Str"("Value"=w412, "Visible"=w413, "Key Focus"=w413, "Text.Selection Start"=u32 0 ("Text.Selection:Start"), "Text.Selection End"=u32 65535 ("Text.Selection:End")) -> ()  [unwired: 2 in, 2 out]
              }
            }
            n329 = property on="SelectRing" class="Ring (strict)"("Visible"=FALSE) -> ()  [unwired: 2 in, 2 out]
          }
          frame 4, 5 {
            n330 = local read "Row"() -> (w418:i32)
            n331 = Index Array(array=w423, index=w418) -> (element=w422:T4)
            n332 = Unbundle By Name(w422) -> ("Device Name"=w419:string, "Sampling Rate (Hz)"=w417:u32, "Bit Depth"=w416:u32)
            n333 = property on="VmaxText" class="Str"("Visible"=FALSE) -> ()  [unwired: 2 in, 2 out]
            n334 = for {
              tunnel: w421 -> [w427] mode=indexing
              tunnel: w419 -> [w428]
              tunnel: w420 -> [w426]
              tunnel: w417 -> [w425]
              tunnel: w416 -> [w424]
              stop <- w429 stop-if-true
              n335 = Unbundle By Name(w427) -> ("Name"=w431:string)
              n336 = Equal?(x=w431, y=w428) -> (x = y?=w430:bool)
              n337 = case shown="True" w430 {
                tunnel: [FALSE TRUE] -> w429
                tunnel: w427 -> [_ w441]
                tunnel: w426 -> [_ w439]
                tunnel: w425 -> [_ w435]
                tunnel: w424 -> [_ w434]
                frame False {
                }
                frame True {
                  n338 = call "CRYGet Freq Bit Array.vi"("Boolean"=FALSE, "Device Infor"=w441) -> ("MinFreq"=w433:u32, "Bit Depth"=w438:cluster{"String":string, "Value":ext}[], "Samplein Rate"=w440:cluster{"String":string, "Value":ext}[])  [unwired: 7 out]
                  n339 = case shown="4" w439 {
                    tunnel: w440 -> [_ w460]
                    tunnel: w438 -> [w442 _]
                    tunnel: w435 -> [_ w458]
                    tunnel: w434 -> [w443 _]
                    tunnel: w433 -> [_ w459]
                    frame 5, Default {
                      n340 = flat-sequence {
                        tunnel: w442 -> [w445]
                        tunnel: w443 -> [w444]
                        tunnel: w442 -> [w455]
                        frame #0 {
                          n341 = for {
                            tunnel: w445 -> [w451] mode=indexing
                            tunnel: w444 -> [w447]
                            stop <- w448 stop-if-true
                            n342 = Unbundle By Name(w451) -> ("Value"=w450:ext)
                            n343 = To Unsigned Long Integer(number=w450) -> (unsigned 32bit integer=w446:u32)
                            n344 = Equal?(x=w446, y=w447) -> (x = y?=w449:bool)
                            n345 = case shown="True" w449 {
                              tunnel: [FALSE TRUE] -> w448
                              tunnel: w447 -> [_ w453]
                              frame False {
                              }
                              frame True {
                                n346 = local write "SelectValue"(w453) -> ()
                              }
                            }
                          }
                        }
                        frame #1 {
                          n347 = local read "SelectValue"() -> (w457:u32)
                          n348 = property on="SelectRing" class="Ring (strict)"("StringsAndValues[]"=w455, "Visible"=TRUE, "Value"=w457) -> ()  [unwired: 2 in, 2 out]
                        }
                      }
                    }
                    frame 4 {
                      n349 = local write "SelectValue"(w459) -> ()
                      n350 = flat-sequence {
                        tunnel: w460 -> [w462]
                        tunnel: w458 -> [w461]
                        tunnel: w460 -> [w472]
                        frame #0 {
                          n351 = for {
                            tunnel: w462 -> [w468] mode=indexing
                            tunnel: w461 -> [w464]
                            stop <- w465 stop-if-true
                            n352 = Unbundle By Name(w468) -> ("Value"=w467:ext)
                            n353 = To Unsigned Long Integer(number=w467) -> (unsigned 32bit integer=w463:u32)
                            n354 = Equal?(x=w463, y=w464) -> (x = y?=w466:bool)
                            n355 = case shown="True" w466 {
                              tunnel: [FALSE TRUE] -> w465
                              tunnel: w464 -> [_ w470]
                              frame False {
                              }
                              frame True {
                                n356 = local write "SelectValue"(w470) -> ()
                              }
                            }
                          }
                        }
                        frame #1 {
                          n357 = local read "SelectValue"() -> (w474:u32)
                          n358 = property on="SelectRing" class="Ring (strict)"("StringsAndValues[]"=w472, "Visible"=TRUE, "Value"=w474) -> ()  [unwired: 2 in, 2 out]
                        }
                      }
                    }
                  }
                }
              }
            }
          }
        }
        n359 = Add(x=w298, y=u32 4) -> (x+y=w295:u32)
        n360 = Bundle("Left"=w306, w305) -> (w301:cluster{"Left":i32, i32})  [unwired: 1 out]
        n361 = Bundle("Width"=w297, w295) -> (w294:cluster{"Width":u32, u32})  [unwired: 1 out]
        n362 = property on="SelectRing" class="Ring (strict)"("Position"=w301, "NmdNumSize"=w299) -> ()  [unwired: 2 in, 2 out]
        n363 = property on="VmaxText" class="Str"("Position"=w301, "Size"=w294) -> ()  [unwired: 2 in, 2 out]
        n364 = local write "SelectSate"(FALSE ("SelectSate")) -> ()
      }
    }
    n365 = Bundle("O_Add"="O_Add", "O_Delete"="O_Delete", "O_Duplicate"="O_Duplicate", "I_Add"="I_Add", "I_Delete"="I_Delete", "I_Duplicate"="I_Duplicate", "Update"="Update") -> (w49:T9)  [unwired: 1 out]
    n366 = Cluster To Array(cluster=w49) -> (array=w50:bool[])
    n367 = Search 1D Array(1D array=w50, element=TRUE) -> (index of element=w58:i32)  [unwired: 1 out]
    n368 = case shown="5" w58 {
      tunnel: w47 -> [_ w92 w112 _ w165 w189 _ _]
      tunnel: "Copy of " ("string") -> [_ _ _ w133 _ _ w211 _]
      frame -1, Default {
      }
      frame 0 {
        # "O_Add"
        n369 = local read "O_Channel Info"() -> (w83:T4[])
        n370 = local read "O_Device Info"() -> (w85:T3)
        n371 = local write "Update"(TRUE ("Update")) -> ()
        n372 = property on="SelectRing" class="Ring (strict)"("Visible"=FALSE) -> ()  [unwired: 2 in, 2 out]
        n373 = property on="VmaxText" class="Str"("Visible"=FALSE) -> ()  [unwired: 2 in, 2 out]
        n374 = Index Array(array=w85, index=0) -> (element=w105:T8)
        n375 = for {
          tunnel: w83 -> [w108] mode=indexing
          tunnel: [w107] -> w84 mode=indexing
          n376 = Unbundle By Name(w108) -> ("Name"=w107:string)
        }
        n377 = Unbundle By Name(w105) -> ("Name"=w96:string, "MaxFreq"=w93:dbl, "Channel"=w99:i32[], "Depths"=w98:i32[])  [unwired: 1 out]
        n378 = Index Array(array=w92, index=0) -> (element=w91:T4)
        n379 = Array Max & Min(array=w98) -> (max value=w94:i32)  [unwired: 3 out]
        n380 = Array Max & Min(array=w99) -> ()  [unwired: 4 out]
        n381 = Divide(x=w93, y=2.0) -> (x/y=w95:dbl)
        n382 = call "CRYMake Not Equal Name.vi"("Name In"="Output Channel Name" ("Name"), "Name array In"=w84) -> ("Name out"=w81:string)  [unwired: 2 in, 7 out]
        n383 = Bundle By Name(cluster=w91, "ID"=0, "Name"=w81, "Digital"=FALSE, "Input"=FALSE, "Device Name"=w96, "Hardware Ch ID"=u8 0, "Vmax (V)"=1.0, "Latency (samples)"=0.0, "Sampling Rate (Hz)"=w93, "Bit Depth"=w94, "Anti-aliasing Factor (%fs)"=w95) -> (w88:T4)
        n384 = Insert Into Array(array=w83, new element=w88) -> (w89:T4[])  [unwired: 1 in]
        n385 = local write "O_Channel Info"(w89) -> ()
      }
      frame 1 {
        # "O_Delete"
        n386 = local read "O_Channel Info"() -> (w113:T4[])
        n387 = local write "Update"(TRUE ("Update")) -> ()
        n388 = property on="SelectRing" class="Ring (strict)"("Visible"=FALSE) -> ()  [unwired: 2 in, 2 out]
        n389 = property on="VmaxText" class="Str"("Visible"=FALSE) -> ()  [unwired: 2 in, 2 out]
        n390 = call "CRYSelect Channel Name Dialog.vi"("Channel Info"=w113, "Out/In Channel"=TRUE) -> ("Selected Channels"=w115:i32[], "Selected Flag"=w114:bool)  [unwired: 2 in, 6 out]
        n391 = case shown="True" w114 {
          tunnel: w115 -> [_ w120]
          tunnel: w113 -> [_ w119]
          tunnel: w112 -> [_ w117]
          frame False {
          }
          frame True {
            n392 = for {
              tunnel: w120 -> [w126]
              tunnel: w119 -> [w121] mode=indexing
              shift-right: [w123] -> w118
              shift-left: w117 -> [w122]
              i -> [w125]
              n393 = Search 1D Array(1D array=w126, element=w125) -> (index of element=w124:i32)  [unwired: 1 out]
              n394 = case shown="0, Default" w124 {
                tunnel: [w127 w130] -> w123
                tunnel: w122 -> [w127 w129]
                tunnel: w121 -> [_ w128]
                frame 0, Default {
                }
                frame -1 {
                  n395 = Insert Into Array(array=w129, new element=w128) -> (w130:T4[])  [unwired: 1 in]
                }
              }
            }
            n396 = local write "O_Channel Info"(w118) -> ()
          }
        }
      }
      frame 2 {
        # "O_Duplicate"
        n397 = local read "O_Channel Info"() -> (w135:T4[])
        n398 = local write "Update"(TRUE ("Update")) -> ()
        n399 = property on="SelectRing" class="Ring (strict)"("Visible"=FALSE) -> ()  [unwired: 2 in, 2 out]
        n400 = property on="VmaxText" class="Str"("Visible"=FALSE) -> ()  [unwired: 2 in, 2 out]
        n401 = call "CRYSelect Channel Name Dialog.vi"("Channel Info"=w135, "Out/In Channel"=TRUE) -> ("Selected Channels"=w137:i32[], "Selected Flag"=w136:bool)  [unwired: 2 in, 6 out]
        n402 = case shown="True" w136 {
          tunnel: w137 -> [_ w143]
          tunnel: w135 -> [_ w141]
          tunnel: w135 -> [_ w139]
          tunnel: w133 -> [_ w140]
          frame False {
          }
          frame True {
            n403 = for {
              tunnel: w143 -> [w154] mode=indexing
              shift-right: [w152] -> w142
              shift-left: w141 -> [w147]
              tunnel: w139 -> [w153]
              tunnel: w140 -> [w148]
              n404 = Index Array(array=w153, index=w154) -> (element=w151:T4)
              n405 = Unbundle By Name(w151) -> ("Name"=w149:string)
              n406 = Concatenate Strings(w148, w149) -> (w145:string)
              n407 = for {
                tunnel: w147 -> [w156] mode=indexing
                tunnel: [w155] -> w146 mode=indexing
                n408 = Unbundle By Name(w156) -> ("Name"=w155:string)
              }
              n409 = call "CRYMake Not Equal Name.vi"("Name In"=w145, "Name array In"=w146) -> ("Name out"=w144:string)  [unwired: 2 in, 7 out]
              n410 = Bundle By Name(cluster=w151, "Name"=w144) -> (w150:T4)
              n411 = Insert Into Array(array=w147, new element=w150) -> (w152:T4[])  [unwired: 1 in]
            }
            n412 = local write "O_Channel Info"(w142) -> ()
          }
        }
      }
      frame 3 {
        # "I_Add"
        n413 = local read "I_Device Info"() -> (w162:T3)
        n414 = local write "Update"(TRUE ("Update")) -> ()
        n415 = property on="SelectRing" class="Ring (strict)"("Visible"=FALSE) -> ()  [unwired: 2 in, 2 out]
        n416 = property on="VmaxText" class="Str"("Visible"=FALSE) -> ()  [unwired: 2 in, 2 out]
        n417 = Index Array(array=w162, index=0) -> (element=w183:T8)
        n418 = Unbundle By Name(w183) -> ("Name"=w174:string, "MaxFreq"=w171:dbl, "Channel"=w177:i32[], "Depths"=w176:i32[])  [unwired: 1 out]
        n419 = Index Array(array=w165, index=0) -> (element=w170:T4)
        n420 = Array Max & Min(array=w176) -> (max value=w172:i32)  [unwired: 3 out]
        n421 = Array Max & Min(array=w177) -> ()  [unwired: 4 out]
        n422 = Divide(x=w171, y=2.0) -> (x/y=w173:dbl)
        n423 = local read "I_Channel Info"() -> (w161:T4[])
        n424 = for {
          tunnel: w161 -> [w186] mode=indexing
          tunnel: [w185] -> w163 mode=indexing
          n425 = Unbundle By Name(w186) -> ("Name"=w185:string)
        }
        n426 = call "CRYMake Not Equal Name.vi"("Name In"="Input Channel Name" ("Name"), "Name array In"=w163) -> ("Name out"=w159:string)  [unwired: 2 in, 7 out]
        n427 = Bundle By Name(cluster=w170, "ID"=0, "Name"=w159, "Digital"=FALSE, "Input"=TRUE, "Device Name"=w174, "Hardware Ch ID"=u8 0, "Vmax (V)"=1.0, "Latency (samples)"=0.0, "Sampling Rate (Hz)"=w171, "Bit Depth"=w172, "Anti-aliasing Factor (%fs)"=w173) -> (w167:T4)
        n428 = Insert Into Array(array=w161, new element=w167) -> (w168:T4[])  [unwired: 1 in]
        n429 = local write "I_Channel Info"(w168) -> ()
      }
      frame 4 {
        # "I_Delete"
        n430 = local read "I_Channel Info"() -> (w191:T4[])
        n431 = property on="SelectRing" class="Ring (strict)"("Visible"=FALSE) -> ()  [unwired: 2 in, 2 out]
        n432 = property on="VmaxText" class="Str"("Visible"=FALSE) -> ()  [unwired: 2 in, 2 out]
        n433 = local write "Update"(TRUE ("Update")) -> ()
        n434 = call "CRYSelect Channel Name Dialog.vi"("Channel Info"=w191, "Out/In Channel"=FALSE) -> ("Selected Channels"=w193:i32[], "Selected Flag"=w192:bool)  [unwired: 2 in, 6 out]
        n435 = case shown="True" w192 {
          tunnel: w193 -> [_ w198]
          tunnel: w191 -> [_ w197]
          tunnel: w189 -> [_ w195]
          frame False {
          }
          frame True {
            n436 = for {
              tunnel: w198 -> [w204]
              tunnel: w197 -> [w199] mode=indexing
              shift-right: [w201] -> w196
              shift-left: w195 -> [w200]
              i -> [w203]
              n437 = Search 1D Array(1D array=w204, element=w203) -> (index of element=w202:i32)  [unwired: 1 out]
              n438 = case shown="0, Default" w202 {
                tunnel: [w205 w208] -> w201
                tunnel: w200 -> [w205 w207]
                tunnel: w199 -> [_ w206]
                frame 0, Default {
                }
                frame -1 {
                  n439 = Insert Into Array(array=w207, new element=w206) -> (w208:T4[])  [unwired: 1 in]
                }
              }
            }
            n440 = local write "I_Channel Info"(w196) -> ()
          }
        }
      }
      frame 5 {
        # "I_Duplicate"
        n441 = local read "I_Channel Info"() -> (w213:T4[])
        n442 = local write "Update"(TRUE ("Update")) -> ()
        n443 = property on="SelectRing" class="Ring (strict)"("Visible"=FALSE) -> ()  [unwired: 2 in, 2 out]
        n444 = property on="VmaxText" class="Str"("Visible"=FALSE) -> ()  [unwired: 2 in, 2 out]
        n445 = call "CRYSelect Channel Name Dialog.vi"("Channel Info"=w213, "Out/In Channel"=FALSE) -> ("Selected Channels"=w215:i32[], "Selected Flag"=w214:bool)  [unwired: 2 in, 6 out]
        n446 = case shown="True" w214 {
          tunnel: w215 -> [_ w221]
          tunnel: w213 -> [_ w219]
          tunnel: w213 -> [_ w217]
          tunnel: w211 -> [_ w218]
          frame False {
          }
          frame True {
            n447 = for {
              tunnel: w221 -> [w232] mode=indexing
              shift-right: [w230] -> w220
              shift-left: w219 -> [w225]
              tunnel: w217 -> [w231]
              tunnel: w218 -> [w226]
              n448 = Index Array(array=w231, index=w232) -> (element=w229:T4)
              n449 = Unbundle By Name(w229) -> ("Name"=w227:string)
              n450 = Concatenate Strings(w226, w227) -> (w223:string)
              n451 = for {
                tunnel: w225 -> [w234] mode=indexing
                tunnel: [w233] -> w224 mode=indexing
                n452 = Unbundle By Name(w234) -> ("Name"=w233:string)
              }
              n453 = call "CRYMake Not Equal Name.vi"("Name In"=w223, "Name array In"=w224) -> ("Name out"=w222:string)  [unwired: 2 in, 7 out]
              n454 = Bundle By Name(cluster=w229, "Name"=w222) -> (w228:T4)
              n455 = Insert Into Array(array=w225, new element=w228) -> (w230:T4[])  [unwired: 1 in]
            }
            n456 = local write "I_Channel Info"(w220) -> ()
          }
        }
      }
      frame 6 {
        n457 = local write "Update"(FALSE ("Update")) -> ()
        n458 = for {
          tunnel: "O_Channel Info" -> [w288] mode=indexing
          tunnel: [w273] -> w236 mode=indexing
          n459 = Unbundle By Name(w288) -> ("Name"=w287:string, "Device Name"=w286:string, "Hardware Ch ID"=w285:u8, "Vmax (V)"=w271:dbl, "Sampling Rate (Hz)"=w282:u32, "Bit Depth"=w281:u32, "Audio Driver"=w269:u16, "ASIOChannel Name"=w268:string)  [unwired: 4 out]
          n460 = Equal To 0?(x=w285) -> (x = 0?=w284:bool)
          n461 = case shown="0, Default" w269 {
            tunnel: w284 -> [_ w293]
            tunnel: [w289 w290] -> w283
            tunnel: w268 -> [w289 _]
            frame 2 {
            }
            frame 0, Default {
              n462 = Select(t="Left" ("Device Name"), s=w293, f="Right" ("Device Name")) -> (s? t:f=w290:string)
            }
          }
          n463 = Format Into String(format string="%#g", w271) -> (resulting string=w270:string)  [unwired: 2 in, 1 out]
          n464 = Number To Decimal String(number=w282) -> (decimal integer string=w278:string)  [unwired: 1 out]
          n465 = Number To Decimal String(number=w281) -> (decimal integer string=w274:string)  [unwired: 1 out]
          n466 = Concatenate Strings(w278, " Hz" ("string")) -> (w276:string)
          n467 = Concatenate Strings(w274, " bit" ("string")) -> (w279:string)
          n468 = Bundle("Name"=w287, "Device Name"=w286, "Device Name"=w283, w270, w276, w279) -> (w275:T10)  [unwired: 1 out]
          n469 = Cluster To Array(cluster=w275) -> (array=w273:string[])
        }
        n470 = for {
          tunnel: "I_Channel Info" -> [w262] mode=indexing
          tunnel: [w245] -> w235 mode=indexing
          n471 = Unbundle By Name(w262) -> ("Name"=w261:string, "Device Name"=w260:string, "Hardware Ch ID"=w259:u8, "Vmax (V)"=w244:dbl, "Latency (samples)"=w247:dbl, "Sampling Rate (Hz)"=w256:u32, "Bit Depth"=w255:u32, "Audio Driver"=w241:u16, "ASIOChannel Name"=w240:string)  [unwired: 3 out]
          n472 = Equal To 0?(x=w259) -> (x = 0?=w258:bool)
          n473 = case shown="2" w241 {
            tunnel: w258 -> [_ w267]
            tunnel: [w263 w264] -> w257
            tunnel: w240 -> [w263 _]
            frame 2 {
            }
            frame 0, Default {
              n474 = Select(t="Left" ("Device Name"), s=w267, f="Right" ("Device Name")) -> (s? t:f=w264:string)
            }
          }
          n475 = Format Into String(format string="%#g", w244) -> (resulting string=w242:string)  [unwired: 2 in, 1 out]
          n476 = Number To Decimal String(number=w256) -> (decimal integer string=w249:string)  [unwired: 1 out]
          n477 = Number To Decimal String(number=w255) -> (decimal integer string=w253:string)  [unwired: 1 out]
          n478 = Number To Decimal String(number=w247) -> (decimal integer string=w246:string)  [unwired: 1 out]
          n479 = Concatenate Strings(w249, " Hz" ("string")) -> (w248:string)
          n480 = Concatenate Strings(w253, " bit" ("string")) -> (w252:string)
          n481 = Bundle("Name"=w261, "Device Name"=w260, "Device Name"=w257, w242, w248, w252, w246) -> (w254:T11)  [unwired: 1 out]
          n482 = Cluster To Array(cluster=w254) -> (array=w245:string[])
        }
        n483 = property on="I_MList" class="MCListbox (strict)"("ItemNames"=w235) -> ()  [unwired: 2 in, 2 out]
        n484 = property on="O_MList" class="MCListbox (strict)"("ItemNames"=w236) -> ()  [unwired: 2 in, 2 out]
      }
    }
    n485 = case shown="True" "OK" {
      tunnel: [w63 w68] -> w21
      tunnel: [w62 w67] -> w20
      frame False {
        n486 = local read "O_Channel Info"() -> (w63:T4[])
        n487 = local read "I_Channel Info"() -> (w62:T4[])
      }
      frame True {
        n488 = local read "O_Channel Info"() -> (w70:T4[])
        n489 = local read "I_Channel Info"() -> (w69:T4[])
        n490 = call "CRYTest IOName Array.vi"("Name In"="I_Name In", "Channel Info In"=w69) -> ("Duplication Flag"=w65:bool, "Name Out"=→"I_Name Out":string[][], "Channel Info Out"=w67:T4[])  [unwired: 7 in]
        n491 = call "CRYTest IOName Array.vi"("Name In"="O_Name In", "Channel Info In"=w70) -> ("Duplication Flag"=w66:bool, "Name Out"=→"O_Name Out":string[][], "Channel Info Out"=w68:T4[])  [unwired: 7 in]
        n492 = Or(x=w65, y=w66) -> (x .or. y?=w64:bool)
        n493 = case shown="True" w64 {
          frame True {
            n494 = call "CRYGet Error Message.vi"("Error No"=8 ("No"), "Kind"="Hardware") -> ("Message"=w75:string, "Window Title"=w76:string)  [unwired: 4 in, 4 out]
            n495 = call "CRYMessage Dialog.vi"("Window Title"=w76, "Message Content"=w75) -> ()  [unwired: 8 in, 2 out]
          }
          frame False {
          }
        }
      }
    }
    n496 = Or(x="OK", y="Cancel") -> (x .or. y?=w61:bool)
  }
  "Return Flag" <- w7
  "I_Channel Info Out" <- w5
  "O_Channel Info Out" <- w6
  n497 = local read "Column"() -> (w1:i32)
  n498 = local read "Row"() -> (w2:i32)
  n499 = local write "Row Old"(w2) -> ()
  n500 = local write "Column Old"(w1) -> ()
